vi "main005_shutter.vi"() -> ()   [LabVIEW 2020]
uses:
  <vilib>/DAQmx/write.llb/DAQmx Write (Analog DBL 1Chan 1Samp).vi
  <vilib>/DAQmx/create/channels.llb/DAQmx Create Channel (AO-Voltage-Basic).vi
  <userlib>/caLab/Private/Put_DBL_PV.vi
panel:
  in  "shutter_invert":bool
  in  "shutter_active?":bool
  in  "shutter_t2":dbl=-1000.0 caption="to [fs]"
  in  "shutter_t1":dbl=-2000.0 caption="from [fs]"
  in  "to Uniblitz":tag="Dev1/ao0"
  in  "Path file to softIOC.dbd":string="C:\\Program Files (x86)\\National Instruments\\LabVIEW 2015\\user.lib\\caLab\\lib"
  out "IOC started":bool=TRUE
  in  "Config File":path=path "T:/trARPES/Labview/Front ends/METIS_delayscan/delayScanEPICS.conf" caption="Soft IOC configuration file"
  in  "Configuration Set":T1(array[cluster])=[{"PV name"="trARPES:DelayStage:t0", "description"="Delay Stage time zero Position", "data type"="ai", "number of elements (waveform only)"=1, "element size (waveform only)"="", []}, {"PV name"="trARPES:DelayStage:p1", "description"="Delay Stage range start", "data type"="ai", "number of elements (waveform only)"=1, "element size (waveform only)"="", []}, {"PV name"="trARPES:DelayStage:p2", "description"="Delay Stage range end", "data type"="ai", "number of elements (waveform only)"=1, "element size (waveform only)"="", []}, {"PV name"="trARPES:DelayStage:Pos", "description"="Current Delay Stage position", "data type"="ai", "number of elements (waveform only)"=1, "element size (waveform only)"="", []}]
  in  "view?":bool
  out "a":waveform(dbl)(graph)={"t0"=timestamp(3671595662.0560446 s since 1904-01-01), "dt"=1.0, "Y"=[-30.78165]}
  out "Waveform Chart":dbl(graph)=5.25341140860948
  out "x*y":dbl=-1720.2895668242609
  in  "to ADC":tag="Dev1/ao1"
  out "DAC error":errorcluster
  out "ESP error":errorcluster
  out "run?":bool
  in  "set_vel":bool
  in  "velocity [fs/s]":dbl=66.71281903963042
  in  "vel_mm":dbl=0.2 caption="velocity [mm/s]"
  out "meas. velocity":dbl
  in  "stop":bool
  out "output voltage":dbl
  in  "start":bool
  in  "go2p1":bool
  out "position [fs]":dbl=-215785.61526054132
  out "position [mm]":dbl=-30.78165
  in  "p2 [mm]":dbl=1.6200981145
  in  "p1 [mm]":dbl=1.4702018855
  in  "interpolate output":bool
  in  "t2 [fs]":dbl=375.58059249108845
  in  "t1 [fs]":dbl=-624.4194075089106
  in  "t0 [mm]":dbl=1.5638
  in  "Axis (1)":i32=3 min=1 max=3
  in  "Serial Link (RS232)":enum16{"RS232", "USB"}(ring)
  in  "VISA resource name":refnum<visa-resource-name>="COM8"
  in  "main_close":bool
  # "Always use CLOSE button to correctly disconnect the device. STOP program afterwards."
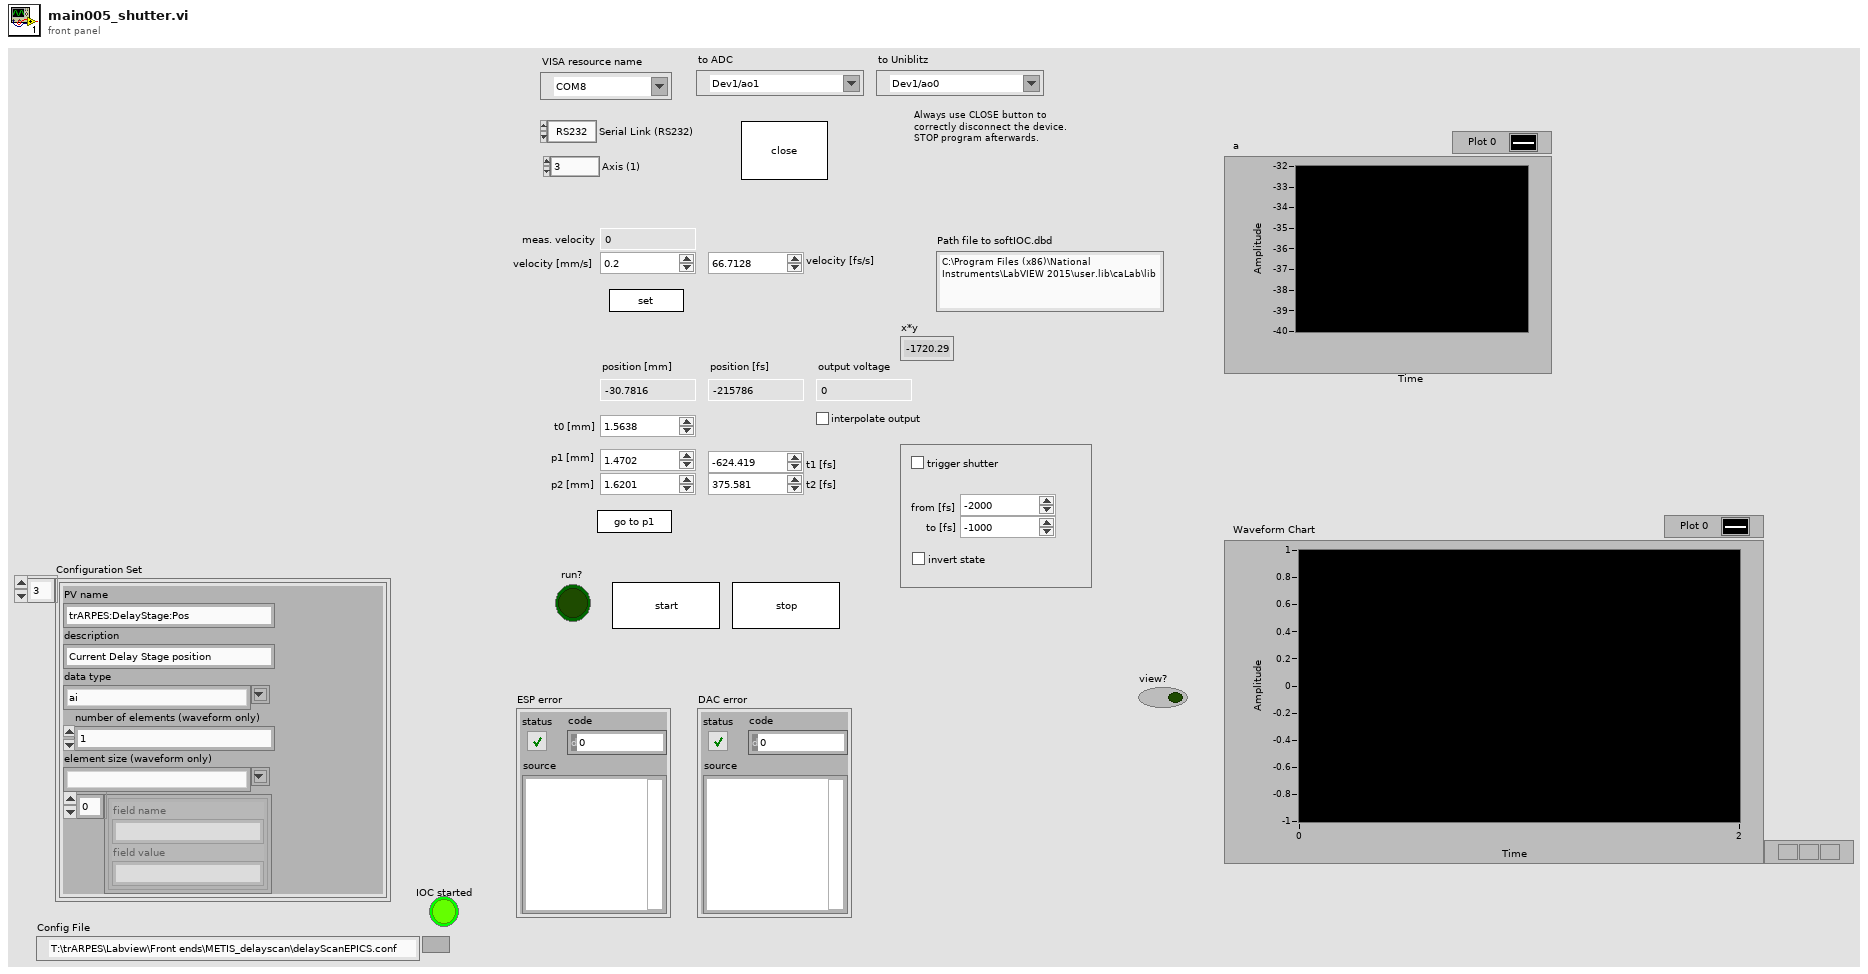
[diagram p1: front panel]
types:
  T1 = cluster{"PV name":string, "description":string, "data type":string, "number of elements (waveform only)":i32, "element size (waveform only)":string, cluster{"field name":string, "field value":string}[]}[]
  T2 = cluster{"dev1_data":refnum<queue>, "dev2_data":refnum<queue>}
  T3 = cluster{"dev1_cmd":refnum<queue>, "dev2_cmd":refnum<queue>}
  T4 = cluster{"PV Name":string, "Data Type":string, "Fields":cluster{"Field Name":string, "Field Value":string}[]}[]
  T5 = cluster{"PV Name":string, "Data Type":string, "Fields":cluster{"Field Name":string, "Field Value":string}[]}
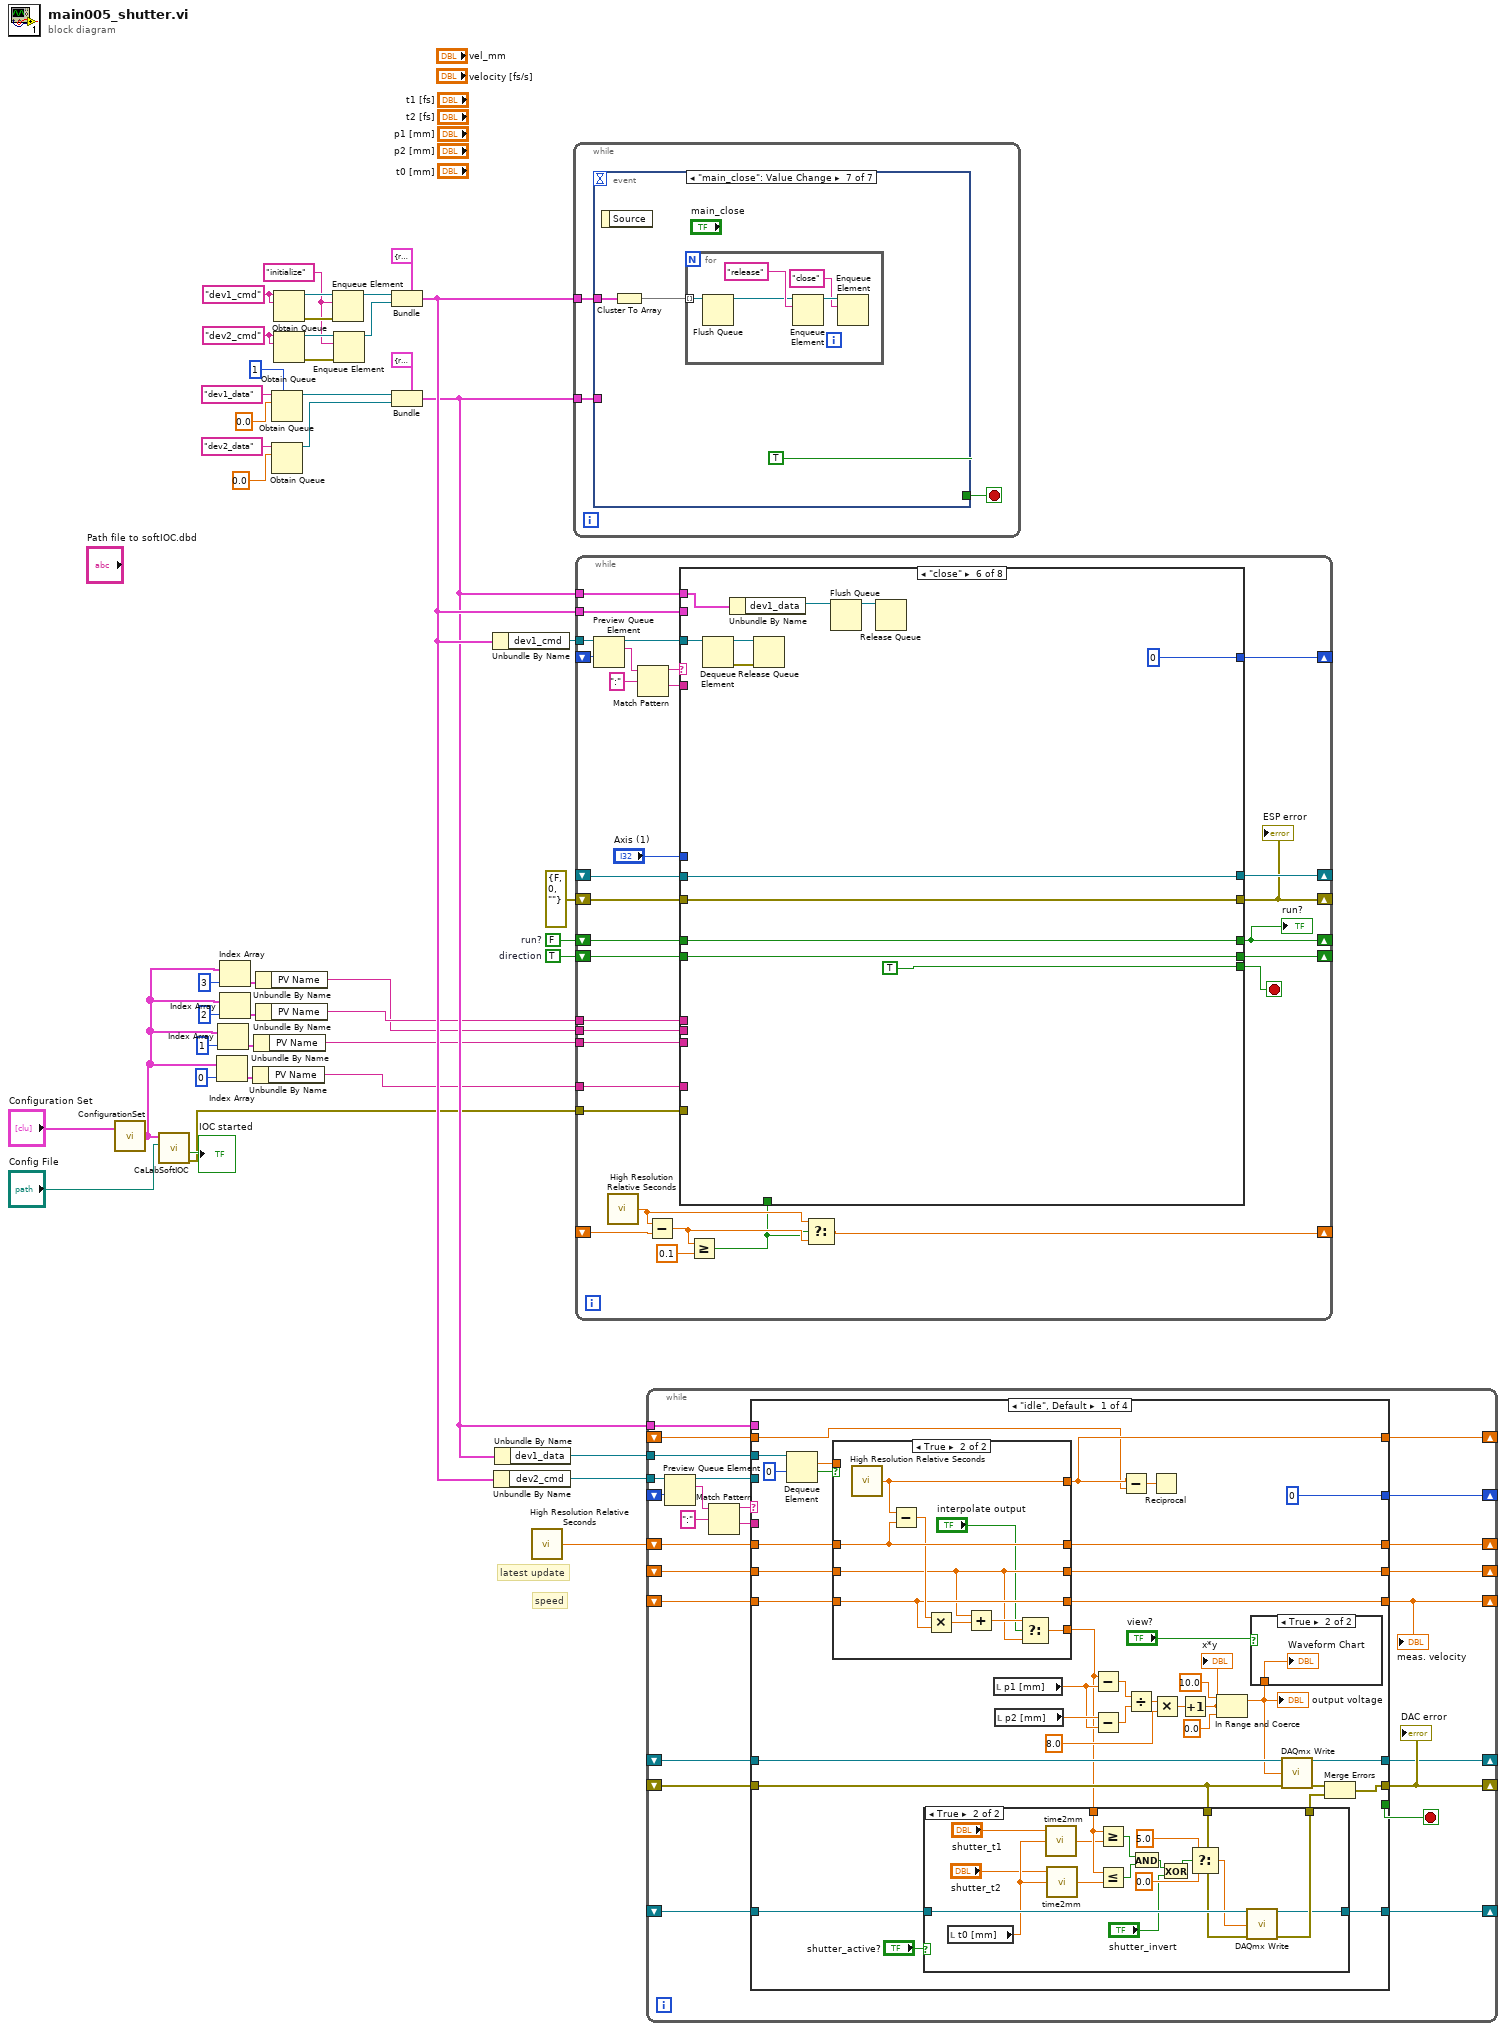
[diagram p0: block diagram]
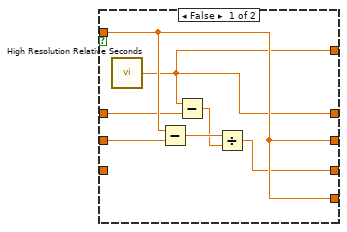
[diagram p4: hidden frame]
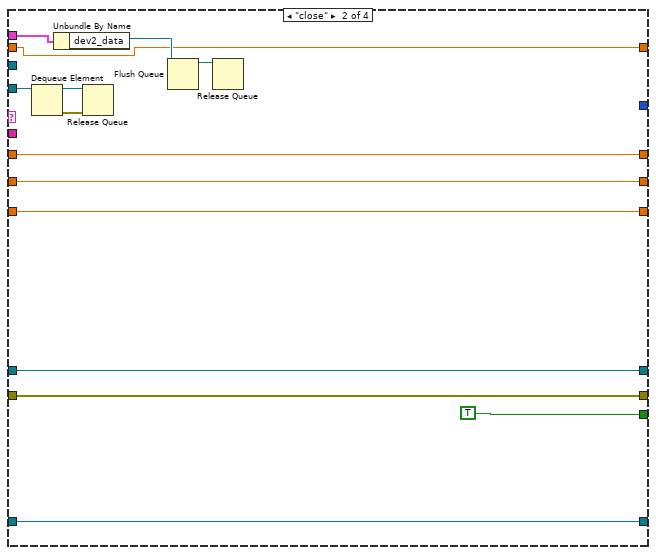
[diagram p5: hidden frame]
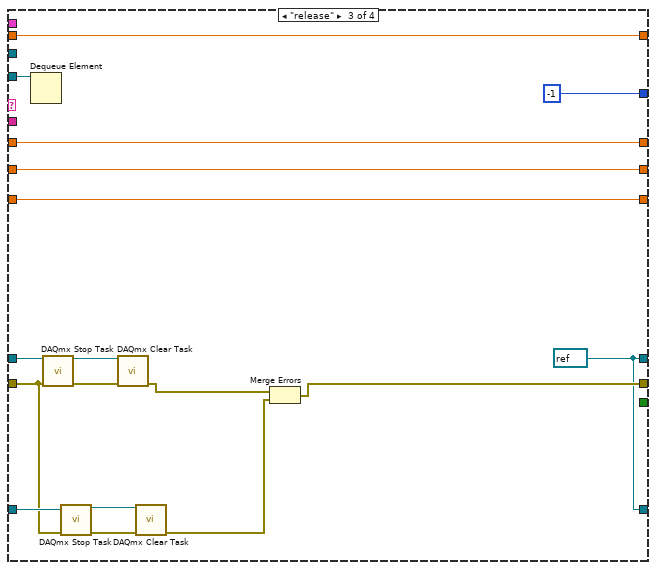
[diagram p6: hidden frame]
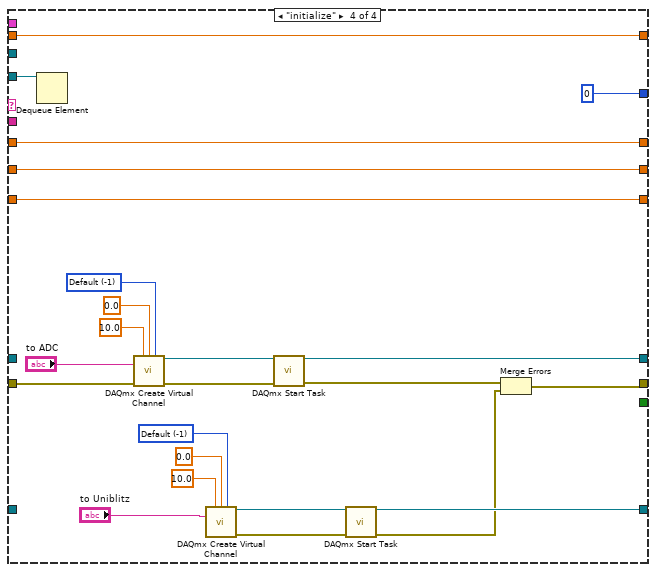
[diagram p7: hidden frame]
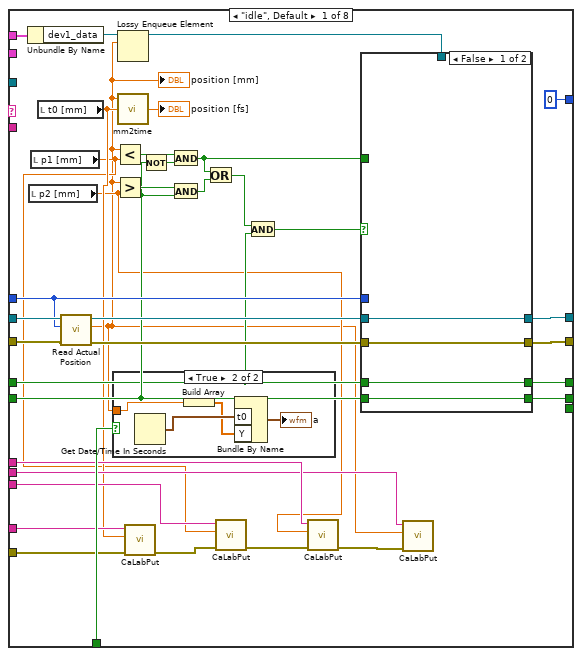
[diagram p8: hidden frame]
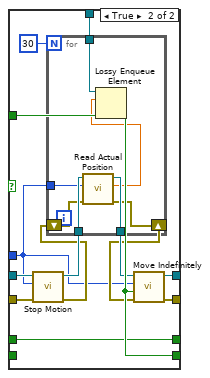
[diagram p10: hidden frame]
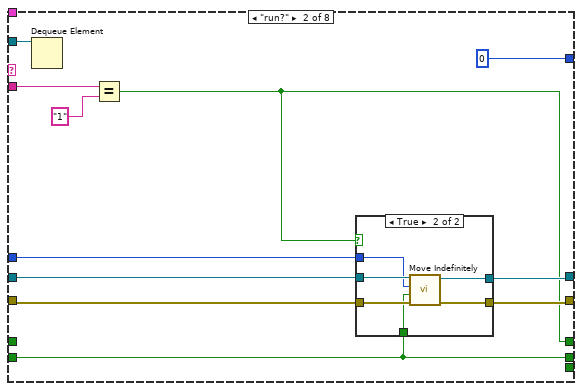
[diagram p11: hidden frame]
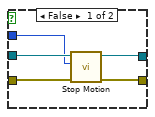
[diagram p12: hidden frame]
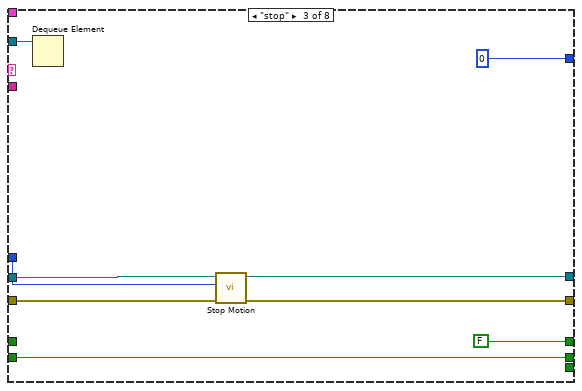
[diagram p13: hidden frame]
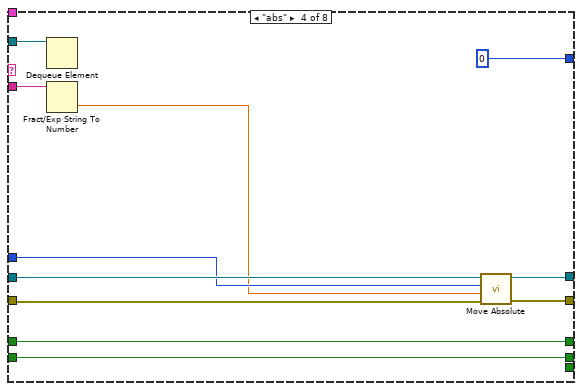
[diagram p14: hidden frame]
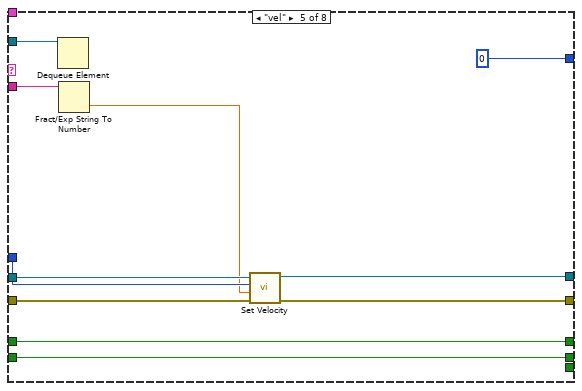
[diagram p15: hidden frame]
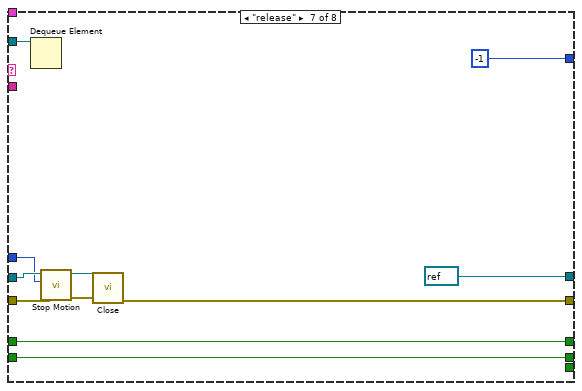
[diagram p16: hidden frame]
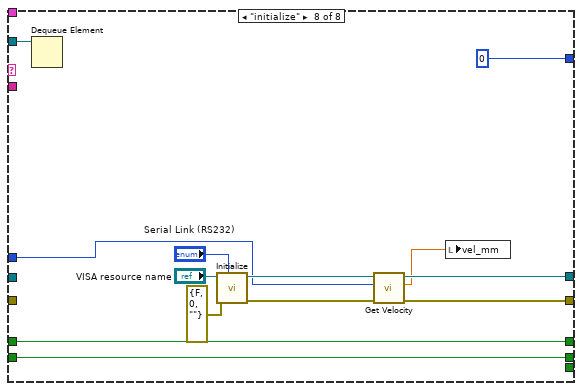
[diagram p17: hidden frame]
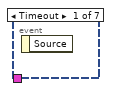
[diagram p18: hidden frame]
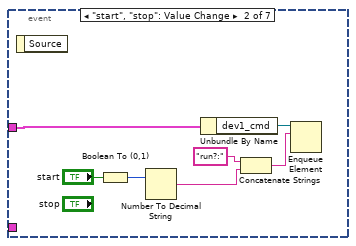
[diagram p19: hidden frame]
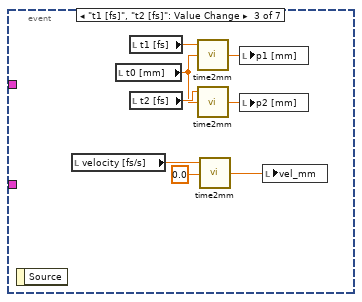
[diagram p20: hidden frame]
diagram:
  w18 = TRUE  # direction
  w21 = FALSE  # run?
  w32 = "dev2_cmd" ("name (unnamed)")
  w38 = "initialize" ("element")
  w33 = "dev1_cmd" ("name (unnamed)")
  # "speed"
  # "latest update"
  n1 = call <userlib>:"ConfigurationSet.vi"("Configuration Set"="Configuration Set") -> ("PV set"=w5:T4)  [unwired: 1 in]
  n2 = call <userlib>:"CaLabSoftIOC.vi"("Config File"="Config File", "PV set"=w5) -> ("error out"=w13:errorcluster, "IOC started"=→"IOC started":bool)  [unwired: 4 in, 2 out]
  n3 = Index Array(array=w5, index=0) -> (element=w16:T5)
  n4 = Index Array(array=w5, index=1) -> (element=w10:T5)
  n5 = Index Array(array=w5, index=3) -> (element=w6:T5)
  n6 = Index Array(array=w5, index=2) -> (element=w9:T5)
  n7 = Unbundle By Name(w16) -> ("PV Name"=w12:string)
  n8 = Unbundle By Name(w10) -> ("PV Name"=w4:string)
  n9 = Unbundle By Name(w6) -> ("PV Name"=w2:string)
  n10 = Unbundle By Name(w9) -> ("PV Name"=w3:string)
  n11 = Obtain Queue(max queue size (-1, unlimited)=1, name (unnamed)="dev1_data", element data type=0.0) -> (queue out=w29:refnum<queue>)  [unwired: 2 in, 2 out]
  n12 = Obtain Queue(name (unnamed)="dev2_data", element data type=0.0) -> (queue out=w28:refnum<queue>)  [unwired: 3 in, 2 out]
  n13 = Obtain Queue(name (unnamed)=w33, element data type=w33) -> (queue out=w44:refnum<queue>, error out=w43:errorcluster)  [unwired: 3 in, 1 out]
  n14 = Obtain Queue(name (unnamed)=w32, element data type=w32) -> (queue out=w39:refnum<queue>, error out=w40:errorcluster)  [unwired: 3 in, 1 out]
  n15 = Enqueue Element(queue=w44, element=w38, error in (no error)=w43) -> (queue out=w41:refnum<queue>)  [unwired: 1 in, 2 out]
  n16 = Enqueue Element(queue=w39, element=w38, error in (no error)=w40) -> (queue out=w37:refnum<queue>)  [unwired: 1 in, 2 out]
  n17 = Bundle(cluster=T3 {"dev1_cmd"=refnum, "dev2_cmd"=refnum}, "dev1_cmd"=w41, "dev2_cmd"=w37) -> (w25:T3)
  n18 = Bundle(cluster=T2 {"dev1_data"=refnum, "dev2_data"=refnum}, "dev1_data"=w29, "dev2_data"=w28) -> (w19:T2)
  n19 = Unbundle By Name(w25) -> ("dev1_cmd"=w34:refnum<queue>)
  n20 = Unbundle By Name(w25) -> ("dev2_cmd"=w24:refnum<queue>)
  n21 = Unbundle By Name(w19) -> ("dev1_data"=w23:refnum<queue>)
  n22 = call <vilib>:"High Resolution Relative Seconds.vi"() -> ("relative seconds"=w22:dbl)
  n23 = while {
    tunnel: w25 -> [w47]
    tunnel: w19 -> [w46]
    stop <- w45 stop-if-true
    n24 = event shown="[6] \"main_close\": Value Change" {
      selector: _ -> [_ _ _ _ _ _ _]
      dyn-events: _ -> [_ _ _ _ _ _ _]
      timeout: _ -> [_ _ _ _ _ _ _]
      tunnel: w47 -> [_ w51 _ w64 _ w82 w85]
      tunnel: w46 -> [_ _ _ _ _ _ _]
      tunnel: [_ _ _ _ _ _ TRUE] -> w45
      event Timeout {
        n25 = event-data() -> ()  [unwired: 1 in, 1 out]
      }
      event "start", "stop": Value Change {
        n26 = event-data() -> ()  [unwired: 1 in, 1 out]
        n27 = Boolean To (0,1)(Boolean="start") -> (0, 1=w49:i16)
        n28 = Number To Decimal String(number=w49) -> (decimal integer string=w48:string)  [unwired: 1 in]
        n29 = Unbundle By Name(w51) -> ("dev1_cmd"=w54:refnum<queue>)
        n30 = Concatenate Strings("run?:" ("string"), w48) -> (w53:string)
        n31 = Enqueue Element(queue=w54, element=w53) -> ()  [unwired: 2 in, 3 out]
      }
      event "t1 [fs]", "t2 [fs]": Value Change {
        n32 = event-data() -> ()  [unwired: 1 in, 1 out]
        n33 = local read "velocity [fs/s]"() -> (w57:dbl)
        n34 = local read "t0 [mm]"() -> (w60:dbl)
        n35 = local read "t1 [fs]"() -> (w61:dbl)
        n36 = local read "t2 [fs]"() -> (w62:dbl)
        n37 = call "time2mm.vi"("Offset (mm)"=w60, "time"=w61) -> ("position (mm)"=w58:dbl)  [unwired: 1 in]
        n38 = call "time2mm.vi"("Offset (mm)"=w60, "time"=w62) -> ("position (mm)"=w59:dbl)  [unwired: 1 in]
        n39 = call "time2mm.vi"("Offset (mm)"=0.0, "time"=w57) -> ("position (mm)"=w55:dbl)  [unwired: 1 in]
        n40 = local write "p1 [mm]"(w58) -> ()
        n41 = local write "p2 [mm]"(w59) -> ()
        n42 = local write "vel_mm"(w55) -> ()
      }
      event "set_vel": Value Change {
        n43 = event-data() -> ()  [unwired: 1 in, 2 out]
        n44 = local read "vel_mm"() -> (w63:dbl)
        n45 = Number To Fractional String(number=w63) -> (F-format string=w67:string)  [unwired: 3 in]
        n46 = Unbundle By Name(w64) -> ("dev1_cmd"=w68:refnum<queue>)
        n47 = Concatenate Strings("vel:" ("string"), w67) -> (w66:string)
        n48 = Enqueue Element(queue=w68, element=w66) -> ()  [unwired: 2 in, 3 out]
      }
      event "p1 [mm]", "p2 [mm]", "t0 [mm]", "vel_mm": Value Change {
        n49 = event-data() -> ()  [unwired: 1 in, 2 out]
        n50 = local read "vel_mm"() -> (w71:dbl)
        n51 = local read "p1 [mm]"() -> (w75:dbl)
        n52 = local read "p2 [mm]"() -> (w76:dbl)
        n53 = local read "t0 [mm]"() -> (w74:dbl)
        n54 = call "mm2time.vi"("Offset (mm)"=w74, "distance (mm)"=w75) -> ("time in fs"=w72:dbl)  [unwired: 1 in]
        n55 = call "mm2time.vi"("Offset (mm)"=w74, "distance (mm)"=w76) -> ("time in fs"=w73:dbl)  [unwired: 1 in]
        n56 = call "mm2time.vi"("Offset (mm)"=0.0, "distance (mm)"=w71) -> ("time in fs"=w70:dbl)  [unwired: 1 in]
        n57 = local write "t1 [fs]"(w72) -> ()
        n58 = local write "t2 [fs]"(w73) -> ()
        n59 = local write "velocity [fs/s]"(w70) -> ()
      }
      event "go2p1": Value Change {
        n60 = event-data() -> ()  [unwired: 1 in, 2 out]
        n61 = local read "p1 [mm]"() -> (w77:dbl)
        n62 = Number To Fractional String(number=w77) -> (F-format string=w80:string)  [unwired: 3 in]
        n63 = Unbundle By Name(w82) -> ("dev1_cmd"=w81:refnum<queue>)
        n64 = Concatenate Strings("abs:" ("string"), w80) -> (w78:string)
        n65 = Enqueue Element(queue=w81, element=w78) -> ()  [unwired: 2 in, 3 out]
      }
      event "main_close": Value Change {
        n66 = event-data() -> ()  [unwired: 1 in, 1 out]
        n67 = Cluster To Array(cluster=w85) -> (array=w84:refnum<queue>[])
        n68 = for {
          tunnel: w84 -> [w90] mode=indexing
          n69 = Flush Queue(queue=w90) -> (queue out=w86:refnum<queue>)  [unwired: 1 in, 2 out]
          n70 = Enqueue Element(queue=w86, element="release") -> (queue out=w88:refnum<queue>)  [unwired: 2 in, 2 out]
          n71 = Enqueue Element(queue=w88, element="close") -> ()  [unwired: 2 in, 3 out]
        }
      }
    }
  }
  n72 = while {
    tunnel: w25 -> [w116]
    tunnel: w34 -> [w121]
    tunnel: w19 -> [w113]
    shift-right: [w111] -> _
    shift-left: _ -> [w112]
    shift-right: [w110] -> _
    shift-left: _ -> [w107]
    shift-right: [w109] -> _
    shift-left: errorcluster {"status"=FALSE, "code"=0, "source"=""} ("error out") -> [w108]
    shift-right: [w104] -> _
    shift-left: w21 -> [w105]
    shift-right: [w102] -> _
    shift-left: w18 -> [w103]
    shift-right: [w96] -> _
    shift-left: _ -> [w101]
    tunnel: w13 -> [w95]
    tunnel: w12 -> [w94]
    tunnel: w4 -> [w93]
    tunnel: w3 -> [w92]
    tunnel: w2 -> [w91]
    stop <- w114 stop-if-true
    n73 = Preview Queue Element(queue=w121, timeout in ms (-1)=w112) -> (queue out=w115:refnum<queue>, element=w120:string)  [unwired: 1 in, 2 out]
    n74 = call <vilib>:"High Resolution Relative Seconds.vi"() -> ("relative seconds"=w98:dbl)
    n75 = Match Pattern(string=w120, regular expression=":") -> (before substring=w118:string, after substring=w117:string)  [unwired: 1 in, 2 out]
    n76 = Subtract(x=w98, y=w101) -> (x-y=w99:dbl)
    n77 = Greater Or Equal?(x=w99, y=0.1) -> (x >= y?=w97:bool)
    n78 = case shown="\"close\"" w118 {
      tunnel: w117 -> [_ w196 _ w226 w233 _ _ _]
      tunnel: w116 -> [_ _ _ _ _ _ _ _]
      tunnel: w115 -> [_ w194 w209 w227 w231 w250 w260 w270]
      tunnel: [_ _ _ _ _ TRUE _ _] -> w114
      tunnel: w113 -> [w156 _ _ _ _ w242 _ _]
      tunnel: [0 0 0 0 0 0 -1 0] -> w111
      tunnel: [w153 w191 w214 w223 w238 w246 refnum<visa-resource-name> refnum ("VISA resource name out") w266] -> w110
      tunnel: [w152 w190 w213 w222 w237 w245 w259 w265] -> w109
      tunnel: w108 -> [w148 w188 w215 w224 w236 w245 w255 _]
      tunnel: w107 -> [w150 w189 w216 w225 w235 w246 w252 _]
      tunnel: "Axis (1)" -> [w149 w192 w212 w221 w234 _ w251 w267]
      tunnel: w105 -> [w137 _ _ w218 w229 w243 w257 w271]
      tunnel: [w136 w187 FALSE ("run?") w218 w229 w243 w257 w271] -> w104
      tunnel: w103 -> [w138 w186 w208 w217 w228 w239 w256 w262]
      tunnel: [w139 w186 w208 w217 w228 w239 w256 w262] -> w102
      tunnel: w97 -> [w135 _ _ _ _ _ _ _]
      tunnel: w95 -> [w133 _ _ _ _ _ _ _]
      tunnel: w94 -> [w129 _ _ _ _ _ _ _]
      tunnel: w93 -> [w128 _ _ _ _ _ _ _]
      tunnel: w92 -> [w127 _ _ _ _ _ _ _]
      tunnel: w91 -> [w126 _ _ _ _ _ _ _]
      frame "idle", Default {
        n79 = Unbundle By Name(w156) -> ("dev1_data"=w155:refnum<queue>)
        n80 = local read "p2 [mm]"() -> (w123:dbl)
        n81 = local read "p1 [mm]"() -> (w124:dbl)
        n82 = local read "t0 [mm]"() -> (w125:dbl)
        n83 = call "Read Actual Position.vi"("error in (no error)"=w148, "Axis (1)"=w149, "VISA resource name"=w150) -> ("error out"=w147:errorcluster, "Position (units)"=w122:dbl, "VISA resource name out"=w146:refnum<visa-resource-name>)  [unwired: 2 in]
        "position [mm]" <- w122
        n84 = case shown="True" w135 {
          tunnel: w122 -> [_ w161]
          frame False {
          }
          frame True {
            n85 = Get Date/Time In Seconds() -> (seconds since 1Jan1904=w160:timestamp)
            n86 = Build Array(w161) -> (w159:dbl[])
            n87 = Bundle By Name("t0"=w160, "Y"=w159) -> (→"a":waveform(dbl))  [unwired: 1 in]
          }
        }
        n88 = Less?(x=w122, y=w124) -> (x < y?=w144:bool)
        n89 = Greater?(x=w122, y=w123) -> (0:w143:bool)
        n90 = Lossy Enqueue Element(queue=w155, element=w122) -> (queue out=w134:refnum<queue>)  [unwired: 1 in, 3 out]
        n91 = call "mm2time.vi"("Offset (mm)"=w125, "distance (mm)"=w122) -> ("time in fs"=→"position [fs]":dbl)  [unwired: 1 in]
        n92 = call-poly <userlib>:"CaLabPut.vi"("Error in (no error)"=w133, "Value"=w125, "PV Name"=w129) -> ("Error out"=w132:errorcluster)  [unwired: 5 in, 3 out]
        n93 = Not(x=w138) -> (.not. x?=w145:bool)
        n94 = And(x=w144, y=w145) -> (x .and. y?=w140:bool)
        n95 = And(x=w143, y=w138) -> (x .and. y?=w142:bool)
        n96 = Or(x=w140, y=w142) -> (x .or. y?=w141:bool)
        n97 = call-poly <userlib>:"CaLabPut.vi"("Error in (no error)"=w132, "Value"=w124, "PV Name"=w128) -> ("Error out"=w131:errorcluster)  [unwired: 5 in, 3 out]
        n98 = And(x=w141, y=w137) -> (x .and. y?=w151:bool)
        n99 = call-poly <userlib>:"CaLabPut.vi"("Error in (no error)"=w131, "Value"=w123, "PV Name"=w127) -> ("Error out"=w130:errorcluster)  [unwired: 5 in, 3 out]
        n100 = case shown="False" w151 {
          tunnel: w146 -> [w165 w176]
          tunnel: w147 -> [w164 w175]
          tunnel: [w165 w178] -> w153
          tunnel: [w164 w177] -> w152
          tunnel: w149 -> [_ w168]
          tunnel: w140 -> [_ w174]
          tunnel: [w163 w174] -> w139
          tunnel: w138 -> [w163 _]
          tunnel: w137 -> [w162 w173]
          tunnel: [w162 w173] -> w136
          tunnel: w134 -> [_ w167]
          frame False {
          }
          frame True {
            n101 = call "Stop Motion.vi"("error in (no error)"=w175, "Axis (1)"=w168, "VISA resource name"=w176) -> ("error out"=w170:errorcluster, "VISA resource name out"=w172:refnum<visa-resource-name>)  [unwired: 3 in]
            n102 = for {
              N: 30 -> [_]
              tunnel: w172 -> [w185]
              tunnel: [w184] -> w171
              shift-right: [w182] -> w169
              shift-left: w170 -> [w183]
              tunnel: w168 -> [w181]
              tunnel: w167 -> [w180]
              n103 = call "Read Actual Position.vi"("error in (no error)"=w183, "Axis (1)"=w181, "VISA resource name"=w185) -> ("error out"=w182:errorcluster, "Position (units)"=w179:dbl, "VISA resource name out"=w184:refnum<visa-resource-name>)  [unwired: 2 in]
              n104 = Lossy Enqueue Element(queue=w180, element=w179) -> ()  [unwired: 1 in, 4 out]
            }
            n105 = call "Move Indefinitely.vi"("error in (no error)"=w169, "Move Direction (+)"=w174, "Axis (1)"=w168, "VISA resource name"=w171) -> ("error out"=w177:errorcluster, "VISA resource name out"=w178:refnum<visa-resource-name>)  [unwired: 2 in]
          }
        }
        n106 = call-poly <userlib>:"CaLabPut.vi"("Error in (no error)"=w130, "Value"=w122, "PV Name"=w126) -> ()  [unwired: 5 in, 4 out]
      }
      frame "run?" {
        n107 = Dequeue Element(queue=w194) -> ()  [unwired: 2 in, 4 out]
        n108 = Equal?(x=w196, y="1") -> (x = y?=w187:bool)
        n109 = case shown="True" w187 {
          tunnel: w189 -> [w201 w207]
          tunnel: w188 -> [w198 w206]
          tunnel: w192 -> [w197 w205]
          tunnel: [w200 w204] -> w191
          tunnel: [w199 w203] -> w190
          tunnel: w186 -> [_ w202]
          frame False {
            n110 = call "Stop Motion.vi"("error in (no error)"=w198, "Axis (1)"=w197, "VISA resource name"=w201) -> ("error out"=w199:errorcluster, "VISA resource name out"=w200:refnum<visa-resource-name>)  [unwired: 3 in]
          }
          frame True {
            n111 = call "Move Indefinitely.vi"("error in (no error)"=w206, "Move Direction (+)"=w202, "Axis (1)"=w205, "VISA resource name"=w207) -> ("error out"=w203:errorcluster, "VISA resource name out"=w204:refnum<visa-resource-name>)  [unwired: 2 in]
          }
        }
      }
      frame "stop" {
        n112 = Dequeue Element(queue=w209) -> ()  [unwired: 2 in, 4 out]
        n113 = call "Stop Motion.vi"("error in (no error)"=w215, "Axis (1)"=w212, "VISA resource name"=w216) -> ("error out"=w213:errorcluster, "VISA resource name out"=w214:refnum<visa-resource-name>)  [unwired: 3 in]
      }
      frame "abs" {
        n114 = Dequeue Element(queue=w227) -> ()  [unwired: 2 in, 4 out]
        n115 = Fract/Exp String To Number(string=w226) -> (number=w220:dbl)  [unwired: 3 in, 1 out]
        n116 = call "Move Absolute.vi"("error in (no error)"=w224, "Position (0 units)"=w220, "Axis (1)"=w221, "VISA resource name"=w225) -> ("error out"=w222:errorcluster, "VISA resource name out"=w223:refnum<visa-resource-name>)  [unwired: 2 in]
      }
      frame "vel" {
        n117 = Dequeue Element(queue=w231) -> ()  [unwired: 2 in, 4 out]
        n118 = Fract/Exp String To Number(string=w233) -> (number=w232:dbl)  [unwired: 3 in, 1 out]
        n119 = call "Set Velocity.vi"("error in (no error)"=w236, "Velocity (units/s)"=w232, "Axis (1)"=w234, "VISA resource name"=w235) -> ("error out"=w237:errorcluster, "VISA resource name out"=w238:refnum<visa-resource-name>)  [unwired: 2 in]
      }
      frame "close" {
        n120 = Dequeue Element(queue=w250) -> (queue out=w249:refnum<queue>, error out=w248:errorcluster)  [unwired: 2 in, 2 out]
        n121 = Unbundle By Name(w242) -> ("dev1_data"=w240:refnum<queue>)
        n122 = Release Queue(queue=w249, error in (no error)=w248) -> ()  [unwired: 1 in, 3 out]
        n123 = Flush Queue(queue=w240) -> (queue out=w241:refnum<queue>)  [unwired: 1 in, 2 out]
        n124 = Release Queue(queue=w241) -> ()  [unwired: 2 in, 3 out]
      }
      frame "release" {
        n125 = Dequeue Element(queue=w260) -> ()  [unwired: 2 in, 4 out]
        n126 = call "Stop Motion.vi"("error in (no error)"=w255, "Axis (1)"=w251, "VISA resource name"=w252) -> ("error out"=w254:errorcluster, "VISA resource name out"=w253:refnum<visa-resource-name>)  [unwired: 3 in]
        n127 = call "Close.vi"("error in (no error)"=w254, "VISA resource name"=w253) -> ("error out"=w259:errorcluster)  [unwired: 9 in]
      }
      frame "initialize" {
        n128 = Dequeue Element(queue=w270) -> ()  [unwired: 2 in, 4 out]
        n129 = call "Initialize.vi"("VISA resource name"="VISA resource name", "error in (no error)"=errorcluster {"status"=FALSE, "code"=0, "source"=""}, "Serial Link (RS232)"="Serial Link (RS232)") -> ("VISA resource name out"=w269:refnum<visa-resource-name>, "error out"=w268:errorcluster)  [unwired: 6 in]
        n130 = call "Get Velocity.vi"("error in (no error)"=w268, "Axis (1)"=w267, "VISA resource name"=w269) -> ("error out"=w265:errorcluster, "Velocity (units/s)"=w264:dbl, "VISA resource name out"=w266:refnum<visa-resource-name>)  [unwired: 2 in]
        n131 = local write "vel_mm"(w264) -> ()
      }
    }
    "run?" <- w104
    "ESP error" <- w109
    n132 = Select(t=w98, s=w97, f=w99) -> (s? t:f=w96:dbl)
  }
  n133 = while {
    shift-right: [w292] -> _
    shift-left: _ -> [w293]
    shift-right: [w291] -> _
    shift-left: _ -> [w290]
    tunnel: w24 -> [w289]
    shift-right: [w288] -> _
    shift-left: _ -> [w287]
    tunnel: w23 -> [w286]
    shift-right: [w285] -> _
    shift-left: _ -> [w282]
    shift-right: [w284] -> _
    shift-left: w22 -> [w283]
    shift-right: [w277] -> _
    shift-left: _ -> [w281]
    tunnel: w19 -> [w280]
    shift-right: [w279] -> _
    shift-left: _ -> [w278]
    shift-right: [w276] -> _
    shift-left: _ -> [w275]
    stop <- w294 stop-if-true
    n134 = Preview Queue Element(queue=w289, timeout in ms (-1)=w293) -> (queue out=w295:refnum<queue>, element=w299:string)  [unwired: 1 in, 2 out]
    n135 = Match Pattern(string=w299, regular expression=":") -> (before substring=w297:string, after substring=w296:string)  [unwired: 1 in, 2 out]
    n136 = case shown="\"idle\", Default" w297 {
      tunnel: w296 -> [_ _ _ _]
      tunnel: w295 -> [_ w386 w402 w420]
      tunnel: [_ TRUE _ _] -> w294
      tunnel: [0 _ -1 0] -> w292
      tunnel: [w304 w382 w388 w404] -> w291
      tunnel: w290 -> [w306 w382 w391 w427]
      tunnel: [w332 w381 w387 w421] -> w288
      tunnel: w287 -> [w331 w381 w401 _]
      tunnel: w286 -> [w333 _ _ _]
      tunnel: [w329 w379 w397 w417] -> w285
      tunnel: [w328 w380 w398 w418] -> w284
      tunnel: w283 -> [w326 w380 w398 w418]
      tunnel: w282 -> [w327 w379 w397 w417]
      tunnel: [w325 w378 w396 w416] -> w277
      tunnel: w281 -> [w324 w378 w396 w416]
      tunnel: w280 -> [_ w375 _ _]
      tunnel: [w314 w374 w395 w414] -> w279
      tunnel: w278 -> [w313 w374 w395 w414]
      tunnel: [w302 w373 w387 w407] -> w276
      tunnel: w275 -> [w307 w373 w392 _]
      frame "idle", Default {
        n137 = Dequeue Element(queue=w333, timeout in ms (-1)=0) -> (element=w330:dbl, timed out?=w315:bool)  [unwired: 1 in, 2 out]
        n138 = case shown="True" w315 {
          tunnel: w330 -> [w363 _]
          tunnel: [w363 w365] -> w300
          tunnel: [w363 w367] -> w329
          tunnel: [w357 w372] -> w328
          tunnel: w327 -> [w362 w367]
          tunnel: w326 -> [w361 w372]
          tunnel: [w358 w369] -> w325
          tunnel: w324 -> [_ w369]
          tunnel: [w357 w364] -> w314
          frame False {
            n139 = call <vilib>:"High Resolution Relative Seconds.vi"() -> ("relative seconds"=w357:dbl)
            n140 = Subtract(x=w363, y=w362) -> (x-y=w360:dbl)
            n141 = Subtract(x=w357, y=w361) -> (x-y=w359:dbl)
            n142 = Divide(x=w360, y=w359) -> (x/y=w358:dbl)
          }
          frame True {
            n143 = call <vilib>:"High Resolution Relative Seconds.vi"() -> ("relative seconds"=w364:dbl)
            n144 = Subtract(x=w364, y=w372) -> (x-y=w371:dbl)
            n145 = Multiply(x=w371, y=w369) -> (x*y=w370:dbl)
            n146 = Add(x=w367, y=w370) -> (x+y=w368:dbl)
            n147 = Select(t=w368, s="interpolate output", f=w367) -> (s? t:f=w365:dbl)
          }
        }
        n148 = case shown="True" "shutter_active?" {
          tunnel: w307 -> [w336 w355]
          tunnel: w306 -> [w337 w354]
          tunnel: [w337 w353] -> w303
          tunnel: [w336 w352] -> w302
          tunnel: w300 -> [_ w351]
          frame False {
          }
          frame True {
            n149 = local read "t0 [mm]"() -> (w343:dbl)
            n150 = call "time2mm.vi"("Offset (mm)"=w343, "time"="shutter_t1") -> ("position (mm)"=w345:dbl)  [unwired: 1 in]
            n151 = call "time2mm.vi"("Offset (mm)"=w343, "time"="shutter_t2") -> ("position (mm)"=w344:dbl)  [unwired: 1 in]
            n152 = Greater Or Equal?(x=w351, y=w345) -> (x >= y?=w349:bool)
            n153 = Less Or Equal?(x=w351, y=w344) -> (x <= y?=w350:bool)
            n154 = And(x=w349, y=w350) -> (x .and. y?=w339:bool)
            n155 = Exclusive Or(1:"shutter_invert", 2:w339) -> (0:w338:bool)
            n156 = Select(t=5.0, s=w338, f=0.0) -> (s? t:f=w348:dbl)
            n157 = call-poly <vilib>:"DAQmx Write.vi"("task/channels in"=w355, "data"=w348, "error in"=w354) -> ("task out"=w352:refnum<k21>, "error out"=w353:errorcluster)  [unwired: 10 in, 1 out]
          }
        }
        n158 = local read "p1 [mm]"() -> (w322:dbl)
        n159 = local read "p2 [mm]"() -> (w323:dbl)
        n160 = Subtract(x=w300, y=w322) -> (x-y=w321:dbl)
        n161 = Subtract(x=w323, y=w322) -> (x-y=w320:dbl)
        n162 = Subtract(x=w314, y=w313) -> (x-y=w312:dbl)
        n163 = Divide(x=w321, y=w320) -> (x/y=w319:dbl)
        n164 = Reciprocal(x=w312) -> ()  [unwired: 1 out]
        n165 = Multiply(x=w319, y=8.0) -> (x*y=w310:dbl)
        n166 = Increment(x=w310) -> (x+1=w309:dbl)
        "x*y" <- w309
        n167 = In Range and Coerce(upper limit=10.0, x=w309, lower limit=0.0) -> (coerced(x)=w311:dbl)  [unwired: 1 out]
        "output voltage" <- w311
        n168 = case shown="True" "view?" {
          tunnel: w311 -> [_ w356]
          frame False {
          }
          frame True {
            "Waveform Chart" <- w356
          }
        }
        n169 = call-poly <vilib>:"DAQmx Write.vi"("task/channels in"=w331, "data"=w311, "error in"=w306) -> ("task out"=w332:refnum<k21>, "error out"=w305:errorcluster)  [unwired: 10 in, 1 out]
        n170 = Merge Errors(w305, w303) -> (w304:errorcluster)
      }
      frame "close" {
        n171 = Dequeue Element(queue=w386) -> (queue out=w385:refnum<queue>, error out=w384:errorcluster)  [unwired: 2 in, 2 out]
        n172 = Unbundle By Name(w375) -> ("dev2_data"=w376:refnum<queue>)
        n173 = Release Queue(queue=w385, error in (no error)=w384) -> ()  [unwired: 1 in, 3 out]
        n174 = Flush Queue(queue=w376) -> (queue out=w377:refnum<queue>)  [unwired: 1 in, 2 out]
        n175 = Release Queue(queue=w377) -> ()  [unwired: 2 in, 3 out]
      }
      frame "release" {
        w387 = refnum<k21> refnum ("task out")
        n176 = Dequeue Element(queue=w402) -> ()  [unwired: 2 in, 4 out]
        n177 = call <vilib>:"DAQmx Stop Task.vi"("task/channels in"=w401, "error in"=w391) -> ("task out"=w400:refnum<k21>, "error out"=w399:errorcluster)  [unwired: 12 in]
        n178 = call <vilib>:"DAQmx Stop Task.vi"("task/channels in"=w392, "error in"=w391) -> ("task out"=w393:refnum<k21>, "error out"=w394:errorcluster)  [unwired: 12 in]
        n179 = call <vilib>:"DAQmx Clear Task.vi"("task in"=w400, "error in"=w399) -> ("error out"=w390:errorcluster)  [unwired: 13 in]
        n180 = call <vilib>:"DAQmx Clear Task.vi"("task in"=w393, "error in"=w394) -> ("error out"=w389:errorcluster)  [unwired: 13 in]
        n181 = Merge Errors(w390, w389) -> (w388:errorcluster)
      }
      frame "initialize" {
        w411 = -1 items=["Default"=-1, "RSE"=10083, "Differential"=10106, "Pseudodifferential"=12529] ("output terminal configuration")
        w424 = -1 items=["Default"=-1, "RSE"=10083, "Differential"=10106, "Pseudodifferential"=12529] ("output terminal configuration")
        n182 = Dequeue Element(queue=w420) -> ()  [unwired: 2 in, 4 out]
        n183 = call-poly <vilib>:"DAQmx Create Virtual Channel.vi"("maximum value"=10.0, "minimum value"=0.0, "output terminal configuration"=w424, "physical channels"="to ADC", "error in"=w427) -> ("task out"=w423:refnum<k21>, "error out"=w422:errorcluster)  [unwired: 9 in]
        n184 = call-poly <vilib>:"DAQmx Create Virtual Channel.vi"("maximum value"=10.0, "minimum value"=0.0, "output terminal configuration"=w411, "physical channels"="to Uniblitz") -> ("task out"=w412:refnum<k21>, "error out"=w413:errorcluster)  [unwired: 10 in]
        n185 = call <vilib>:"DAQmx Start Task.vi"("task/channels in"=w423, "error in"=w422) -> ("task out"=w421:refnum<k21>, "error out"=w406:errorcluster)  [unwired: 12 in]
        n186 = call <vilib>:"DAQmx Start Task.vi"("task/channels in"=w412, "error in"=w413) -> ("task out"=w407:refnum<k21>, "error out"=w405:errorcluster)  [unwired: 12 in]
        n187 = Merge Errors(w406, w405) -> (w404:errorcluster)
      }
    }
    "meas. velocity" <- w277
    "DAC error" <- w291
  }
